vi "Read Direction.vi"(8 "error in (no error)":errorcluster, 11 "Attack in":refnum<class "Net Attack.lvclass">) -> (0 "error out":errorcluster, 2 "Direction":T1, 3 "Attack out":refnum<class "Net Attack.lvclass">)   [LabVIEW 2015, in "Net Attack.lvclass"]
uses:
  Net Attack.lvclass
  Type Defs/Direction Enum.ctl
  Square/Square.lvclass
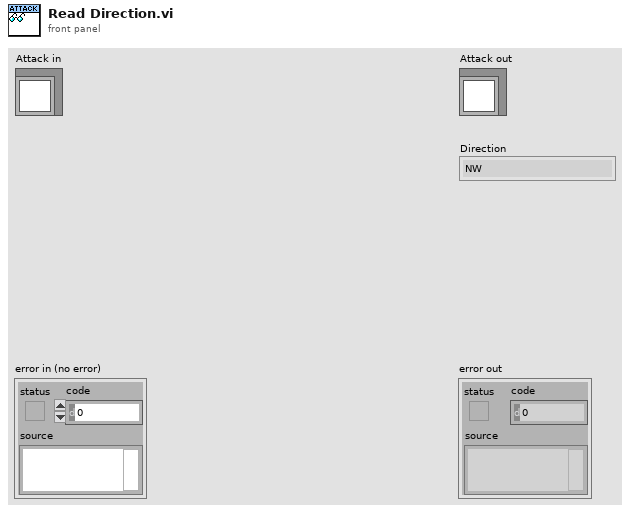
[diagram p1: front panel]
types:
  T1 = typedef "Square.lvclass/Direction Enum.ctl" = enum16{"NW", "N", "NE", "E", "SE", "S", "SW", "W"}
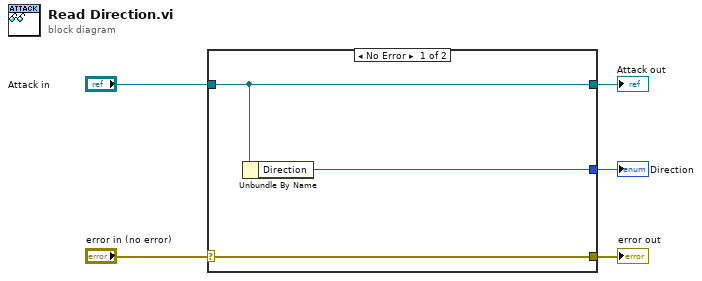
[diagram p0: block diagram]
diagram:
  n1 = case shown="No Error" "error in (no error)" {
    selector: "error in (no error)" -> [w8 w9]
    tunnel: [w8 w9] -> w4
    tunnel: [w7 w10] -> w2
    tunnel: "Attack in" -> [w7 w10]
    tunnel: [w6 _] -> w1
    frame No Error {
      n2 = Unbundle By Name(w7) -> ("Direction"=w6:T1)
    }
    frame Error {
    }
  }
  "error out" <- w4
  "Attack out" <- w2
  "Direction" <- w1
